vi "FFT Globals.vi"() -> ()   [LabVIEW 2023, in "FFT.lvlib" / "FFT.lvclass"]
uses:
  FFT.lvclass
panel:
  in  "Number of FFT Samples":string="Number of FFT Samples"
  in  "Filter":string="Filter"
  in  "Select Channels":string="Select Channels"
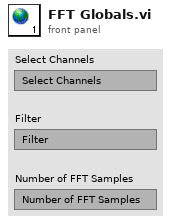
[diagram p1: front panel]
diagram:
